vi "SensitivityV2.vi"(9 "Min Output":dbl(slide) scale=0.0..1.0, 10 "Max Output":dbl(slide) scale=0.0..1.0, 11 "Points":dbl[][](array[slide]) scale=0.0..1.0) -> (2 "Yi":dbl[](array[numeric]) format="%_6g", 3 "XY Graph":cluster{dbl[], dbl[]}[](graph))   [LabVIEW 2017]
uses:
  <vilib>/Analysis/1siggen.llb/Ramp Pattern by Delta.vi
  <vilib>/gmath/NI_Gmath.lvlib
  <vilib>/Analysis/NI_AALBase.lvlib
panel:
  out "Points":dbl[][](array[numeric])
  in  "# of Points":i8 min=0 max=10
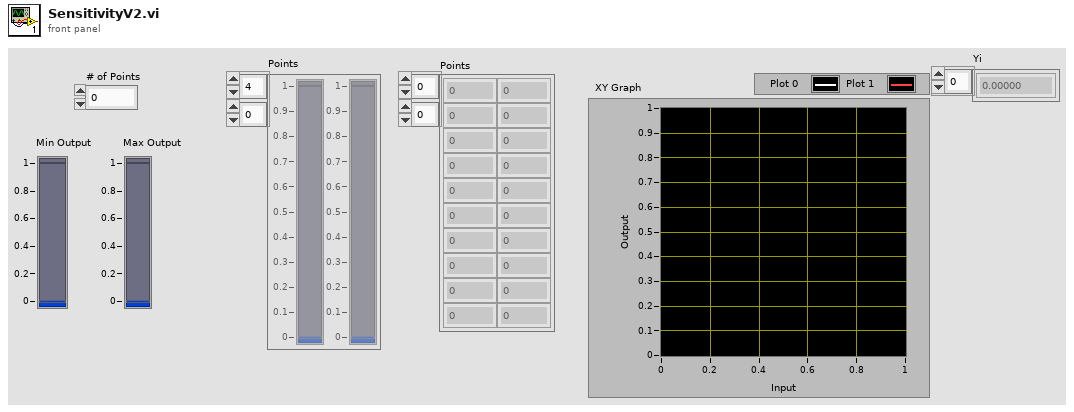
[diagram p1: front panel]
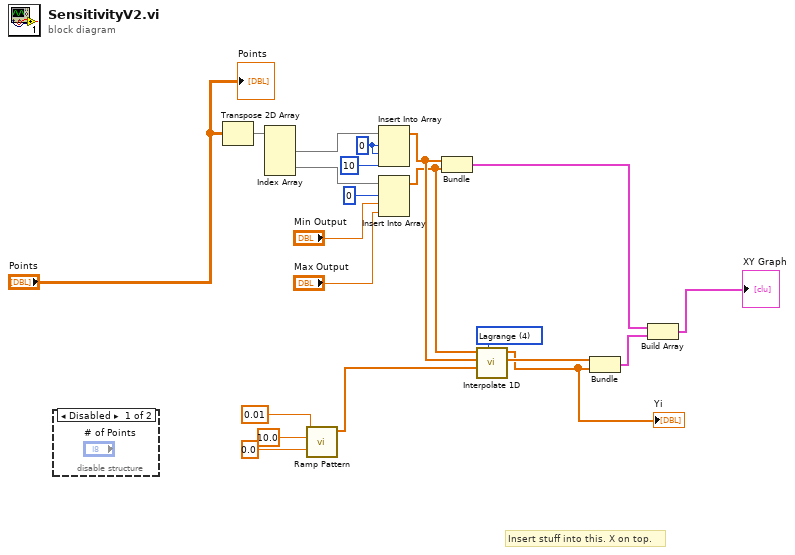
[diagram p0: block diagram]
diagram:
  w11 = 0 ("index")
  w18 = 4 items=["nearest", "linear", "spline", "cubic Hermite", "Lagrange"] ("method")
  # "Insert stuff into this. X on top."
  n1 = disable-structure shown="Disabled" {
    frame Disabled {
    }
    frame Enabled {
    }
  }
  n2 = Transpose 2D Array(2D array="Points") -> (transposed array=w21:dbl[][])
  n3 = Index Array(array=w21) -> (element #1=w12:dbl[], element #2=w14:dbl[])  [unwired: 4 in]
  n4 = call-poly <vilib>:"Ramp Pattern.vi"("start"=0.0, "end"=10.0, "delta"=0.01) -> ("Ramp Pattern"=w15:dbl[])  [unwired: 6 in, 2 out]
  n5 = Insert Into Array(array=w12, index=w11, new element #1=w11, new element #2=10 ("index")) -> (w10:dbl[])
  n6 = Insert Into Array(array=w14, index=0, new element #1="Min Output", new element #2="Max Output") -> (w9:dbl[])
  n7 = Bundle(w10, w9) -> (w8:cluster{dbl[], dbl[]})  [unwired: 1 in]
  n8 = call <vilib>:"Interpolate 1D.vi"("method"=w18, "xi"=w15, "X"=w10, "Y"=w9) -> ("xi used"=w3:dbl[], "yi"=w1:dbl[])  [unwired: 5 in, 1 out]
  "Yi" <- w1
  n9 = Bundle("xi used"=w3, "yi"=w1) -> (w19:cluster{"xi used":dbl[], "yi":dbl[]})  [unwired: 1 in]
  n10 = Build Array(w8, w19) -> (→"XY Graph":cluster{"xi used":dbl[], "yi":dbl[]}[])
  "Points" <- "Points"
